vi "ReciveLine.vi"(8 "error in (no error)":errorcluster caption="Fehler (Eingang, kein Fehler)", 11 "MoveoSerial Eingang":refnum<class "MoveoSerial.lvclass">) -> (0 "error out":errorcluster caption="Fehler (Ausgang)", 3 "MoveoSerial Ausgang":refnum<class "MoveoSerial.lvclass">)   [LabVIEW 2019, in "MoveoSerial.lvclass"]
uses:
  MoveoSerial.lvclass
  MoveoSerial.lvclass/MoveoSerial.ctl
panel:
  out "Bytes at Port":bool
  out "Schreibpuffer":string
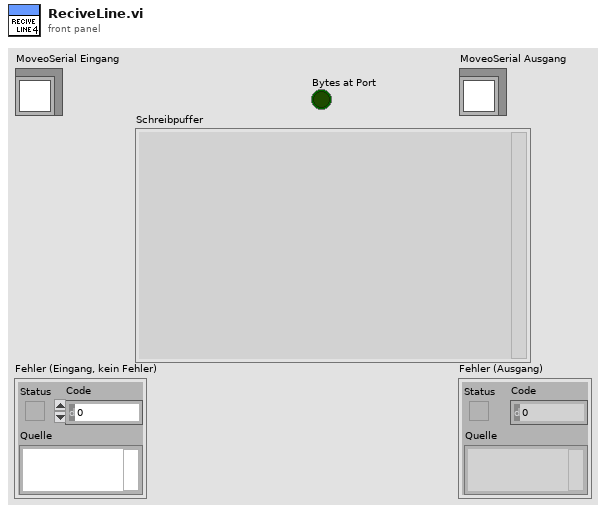
[diagram p1: front panel]
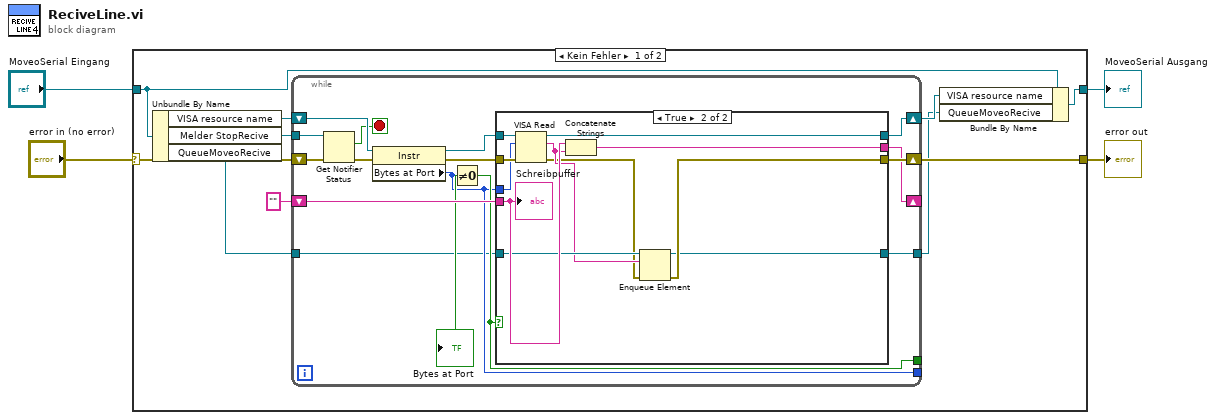
[diagram p0: block diagram]
diagram:
  n1 = case shown="Kein Fehler" "error in (no error)" {
    selector: "error in (no error)" -> [w13 w46]
    tunnel: [w12 w46] -> w3
    tunnel: [w9 w45] -> w1
    tunnel: "MoveoSerial Eingang" -> [w10 w45]
    frame No Error {
      n2 = Unbundle By Name(w10) -> ("VISA resource name"=w14:refnum<visa-resource-name>, "Melder StopRecive"=w7:refnum<notifier>, "QueueMoveoRecive"=w6:refnum<queue>)
      n3 = while {
        tunnel: [w25] -> _
        shift-right: [w29] -> w8
        shift-left: w14 -> [w23]
        shift-right: [w28] -> w12
        shift-left: w13 -> [w19]
        shift-right: [w26] -> _
        shift-left: "" -> [w27]
        tunnel: [w24] -> _
        tunnel: w7 -> [w20]
        tunnel: w6 -> [w16]
        tunnel: [w15] -> w5
        stop <- w17 stop-if-true
        n4 = Get Notifier Status(notifier=w20, error in (no error)=w19) -> (current notification=w17:bool, error out=w18:errorcluster)  [unwired: 3 out]
        n5 = property class="Instr"(reference=w23, error in=w18) -> (reference out=w22:refnum<visa-resource-name>, error out=w21:errorcluster, "Bytes at Port"=w24:u32)
        n6 = Not Equal To 0?(x=w24) -> (x != 0?=w25:bool)
        "Bytes at Port" <- w25
        n7 = case shown="True" w25 {
          tunnel: w22 -> [w33 w44]
          tunnel: w21 -> [w32 w43]
          tunnel: [w33 w42] -> w29
          tunnel: [w32 w35] -> w28
          tunnel: w27 -> [w31 w41]
          tunnel: [w31 w40] -> w26
          tunnel: w24 -> [_ w39]
          tunnel: w16 -> [w30 w38]
          tunnel: [w30 w34] -> w15
          frame False {
          }
          frame True {
            n8 = VISA Read(VISA resource name=w44, byte count=w39, error in (no error)=w43) -> (VISA resource name out=w42:refnum<visa-resource-name>, read buffer=w37:string, error out=w36:errorcluster)  [unwired: 1 out]
            n9 = Concatenate Strings(w41, w37) -> (w40:string)
            n10 = Enqueue Element(queue=w38, element=w37, error in (no error)=w36) -> (queue out=w34:refnum<queue>, error out=w35:errorcluster)  [unwired: 1 in, 1 out]
            "Schreibpuffer" <- w41
          }
        }
      }
      n11 = Bundle By Name(cluster=w10, "VISA resource name"=w8, "QueueMoveoRecive"=w5) -> (w9:refnum<class "MoveoSerial.lvclass">)
    }
    frame Error {
    }
  }
  "error out" <- w3
  "MoveoSerial Ausgang" <- w1
